vi "Determine Acc Angle.vi"(8 "za":dbl[](array[numeric]), 9 "ya":dbl[](array[numeric]), 10 "xa":dbl[](array[numeric]), 11 "Acc":dbl[][](array[numeric])) -> (0 "z scale":dbl, 1 "yscale":dbl, 2 "xscale":dbl, 3 "output angle":dbl[](array[numeric]))   [LabVIEW 2015]
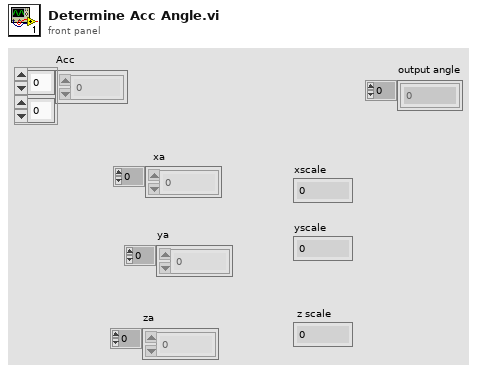
[diagram p1: front panel]
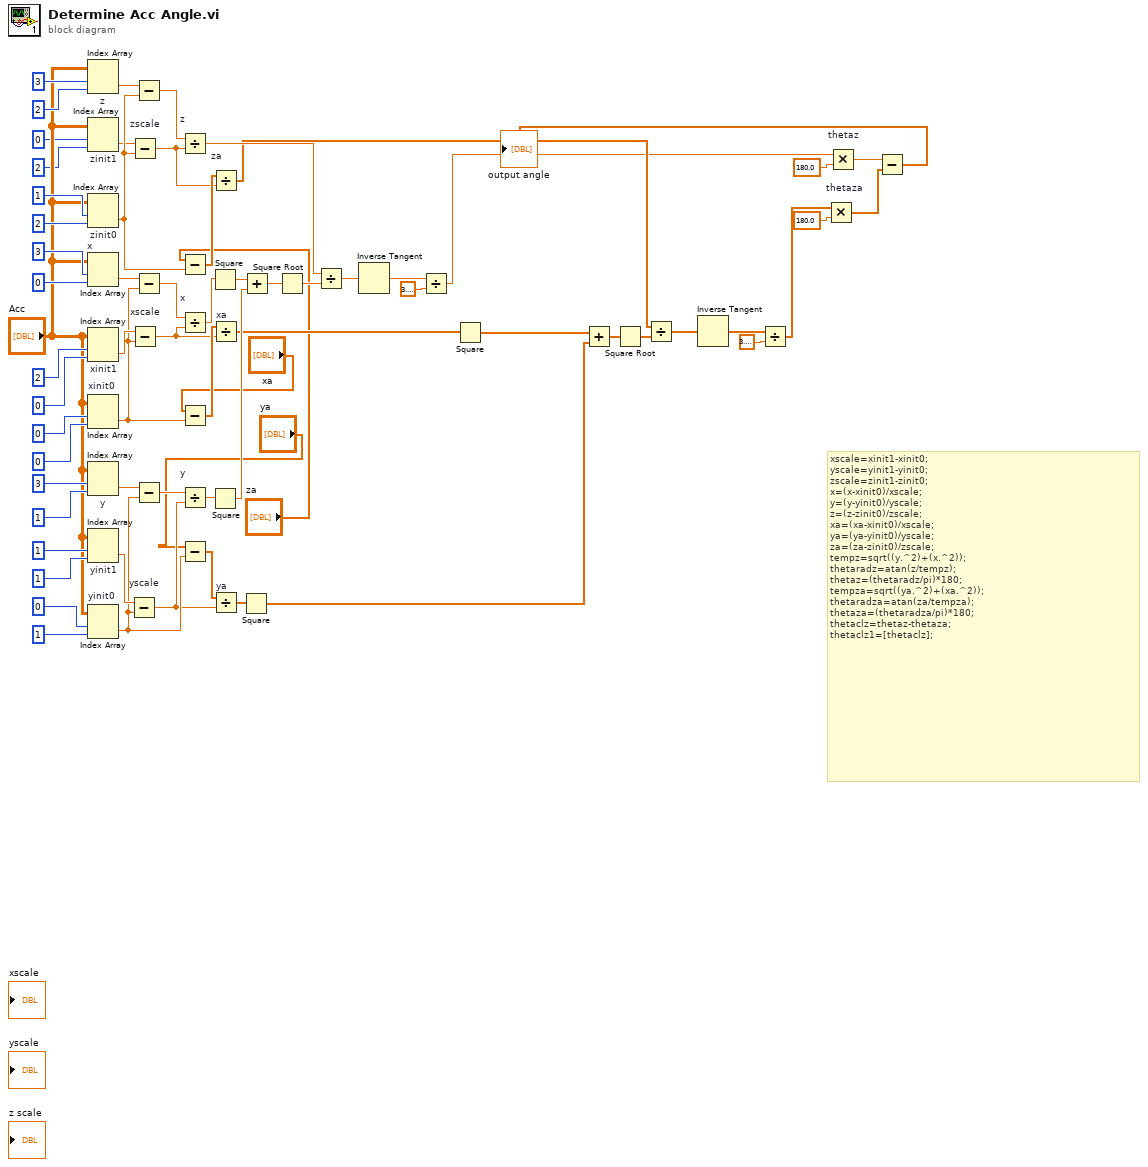
[diagram p0: block diagram]
diagram:
  # "xscale=xinit1-xinit0;\nyscale=yinit1-yinit0;\nzscale=zinit1-zinit0;\nx=(x-xinit0)/xscale;\ny=(y-yinit0)/yscale;\nz=(z-zinit0)/zscale;\nxa=(xa-xinit0)/xscale;\nya=(ya-yinit0)/yscale;\nza=(za-zinit0)/zscale;\ntempz=sqrt((y.^2)+(x.^2));\nthetaradz=atan(z/tempz);\nthetaz=(thetaradz/pi)*180;\ntempza=sqrt((ya.^2)+(xa.^2));\nthetaradza=atan(za/tempza);\nthetaza=(thetaradza/pi)*180;\nthetaclz=thetaz-thetaza;\nthetaclz1=[thetaclz];"
  n1 = Index Array "z"(array="Acc", index (row)=3, index (col)=2 ("disabled index (col)")) -> (element=w43:dbl)
  n2 = Index Array "zinit1"(array="Acc", index (row)=0, index (col)=2 ("disabled index (col)")) -> (element=w6:dbl)
  n3 = Index Array "zinit0"(array="Acc", index (row)=1, index (col)=2) -> (element=w7:dbl)
  n4 = Index Array "x"(array="Acc", index (row)=3, index (col)=0 ("disabled index (col)")) -> (element=w46:dbl)
  n5 = Index Array "xinit1"(array="Acc", index (row)=2, index (col)=0 ("disabled index (col)")) -> (element=w48:dbl)
  n6 = Index Array "xinit0"(array="Acc", index (row)=0, index (col)=0 ("disabled index (col)")) -> (element=w5:dbl)
  n7 = Index Array "y"(array="Acc", index (row)=3, index (col)=1 ("disabled index (col)")) -> (element=w44:dbl)
  n8 = Index Array "yinit1"(array="Acc", index (row)=1, index (col)=1 ("disabled index (col)")) -> (element=w47:dbl)
  n9 = Index Array "yinit0"(array="Acc", index (row)=0, index (col)=1) -> (element=w40:dbl)
  n10 = Subtract "yscale"(x=w47, y=w40) -> (x-y=w10:dbl)
  n11 = Subtract "zscale"(x=w6, y=w7) -> (x-y=w8:dbl)
  n12 = Subtract "xscale"(x=w48, y=w5) -> (x-y=w9:dbl)
  n13 = Subtract(x=w43, y=w7) -> (x-y=w41:dbl)
  n14 = Subtract(x=w46, y=w5) -> (x-y=w45:dbl)
  n15 = Subtract(x=w44, y=w40) -> (x-y=w42:dbl)
  n16 = Divide "z"(x=w41, y=w8) -> (x/y=w30:dbl)
  n17 = Subtract(x="za", y=w7) -> (x-y=w39:dbl[])
  n18 = Divide "x"(x=w45, y=w9) -> (x/y=w36:dbl)
  n19 = Subtract(x="xa", y=w5) -> (x-y=w38:dbl[])
  n20 = Divide "y"(x=w42, y=w10) -> (x/y=w35:dbl)
  n21 = Subtract(x="ya", y=w40) -> (x-y=w37:dbl[])
  n22 = Square(x=w36) -> (x^2=w34:dbl)
  n23 = Square(x=w35) -> (x^2=w33:dbl)
  n24 = Divide "za"(x=w39, y=w8) -> (x/y=w21:dbl[])
  n25 = Divide "xa"(x=w38, y=w9) -> (x/y=w27:dbl[])
  n26 = Divide "ya"(x=w37, y=w10) -> (x/y=w26:dbl[])
  n27 = Square(x=w26) -> (x^2=w24:dbl[])
  n28 = Add(x=w34, y=w33) -> (x+y=w32:dbl)
  n29 = Square Root(x=w32) -> (sqrt(x)=w31:dbl)
  n30 = Divide(x=w30, y=w31) -> (x/y=w29:dbl)
  n31 = Inverse Tangent(1:w29) -> (0:w15:dbl)
  n32 = Divide(x=w15, y=3.141592653589793) -> (x/y=w13:dbl)
  n33 = Square(x=w27) -> (x^2=w25:dbl[])
  n34 = Add(x=w25, y=w24) -> (x+y=w23:dbl[])
  n35 = Square Root(x=w23) -> (sqrt(x)=w22:dbl[])
  n36 = Divide(x=w21, y=w22) -> (x/y=w20:dbl[])
  n37 = Inverse Tangent(1:w20) -> (0:w11:dbl[])
  n38 = Divide(x=w11, y=3.141592653589793) -> (x/y=w19:dbl[])
  n39 = Multiply "thetaza"(x=w19, y=180.0) -> (x*y=w16:dbl[])
  n40 = Multiply "thetaz"(x=w13, y=180.0) -> (x*y=w17:dbl)
  n41 = Subtract(x=w17, y=w16) -> (x-y=→"output angle":dbl[])
